vi "multiSineRT_inst.vi"() -> ()   [LabVIEW 2019]
uses:
  <vilib>/myRIO/Common/Instrument Driver Framework/myRIO v1.0/IRQ/typedefs/DI IRQ Type.ctl
  <vilib>/userDefined/High Color/nirio_resource_hc.ctl
  <vilib>/Platform/TimedLoop/XDataNode/timing_clust.ctl
  <vilib>/Platform/TimedLoop/XDataNode/nitl_modes.ctl
  <vilib>/Platform/TimedLoop/XDataNode/wakeup.ctl
  <vilib>/Utility/file.llb/Read Delimited Spreadsheet (DBL).vi
  rpm.vi
  ISR.vi
  <vilib>/myRIO/Common/Instrument Driver Framework/myRIO v1.0/IRQ/vis/myRIO v1.1 Register DI IRQ.vi
  <vilib>/Utility/file.llb/Write Delimited Spreadsheet (DBL).vi
  <vilib>/Utility/error.llb/Error Cluster From Error Code.vi
  <vilib>/myRIO/Common/Instrument Driver Framework/myRIO v1.0/PWM/vis/myRIO v1.0 Write PWM.vi
  <vilib>/myRIO/Common/Instrument Driver Framework/myRIO v1.0/IRQ/vis/myRIO v1.0 Reserve IRQ.vi
  <vilib>/myRIO/Common/Instrument Driver Framework/Utilities/vis/FPGA Ref Manager.vi
  <vilib>/myRIO/Common/Instrument Driver Framework/myRIO v1.0/myRIO v1.0 Close.vi
  <vilib>/myRIO/Express VI/IRQ/IRQ Express VI.xnode
  <vilib>/myRIO/Instrument Drivers/IRQ/IO IRQ/vis/myRIO Register DI IRQ.xnode
  <vilib>/myRIO/Common/Instrument Driver Framework/myRIO v1.0/IRQ/typedefs/Callback VI Ref.ctl
  <vilib>/platform/TimedLoop/XDataNode/XDataNode.xnode
  <vilib>/Platform/TimedLoop/XDataNode/XDNodeRunTimeDep.lvlib
  <vilib>/myRIO/Instrument Drivers/Onboard IO/PWM/PWM.lvlib
  <vilib>/Utility/Variable/NI_VariableUtilities.lvlib
  <vilib>/myRIO/Instrument Drivers/IRQ/IO IRQ/IO IRQ.lvlib
panel:
  out "g_p":dbl
  out "k_p":dbl
  out "error out (no error) 2":errorcluster
  out "p":dbl
  out "Commutations":i64
  out "RPM":dbl
  out "Iteration Duration":i64
  out "omega_vec":dbl[](array[numeric])
  out "Interrupt On":bool
  in  "RPM Inst Data":path=path "/tmp/log.csv"
  out "Omega":dbl[](graph)
  in  "error in (no error)":errorcluster
  out "Np":dbl
  out "ft":dbl
  in  "Input Data":path=path "/tmp/log.csv"
  in  "del_u":dbl=0.15
  in  "u_nominal":dbl=0.55
  out "Finished late":bool
  out "Acquisition State":bool
  in  "Run Time (s)":dbl
  in  "Sampling \nFrequency (Hz)":dbl
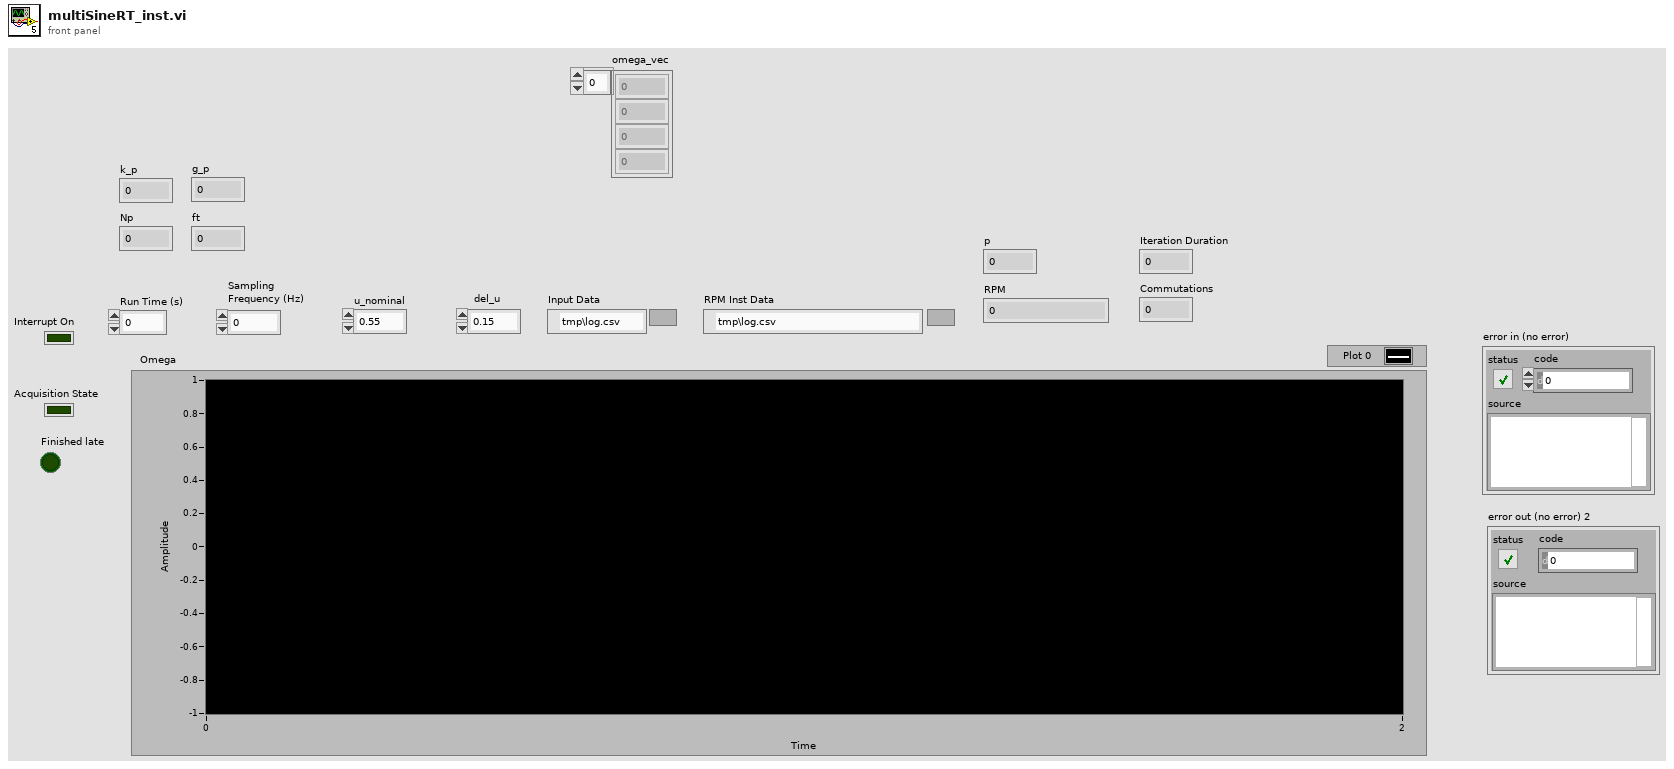
[diagram p1: front panel]
types:
  T1 = typedef "PWM.lvlib/PWM Reference.ctl" = cluster{"myRIO Reference":T2, "PWM Channels Enum":T6, "PWM Configuration":T7}
  T2 = typedef "myRIO Generic Hardware Reference.ctl" = cluster{"myRIO Model":T3, "myRIO Hardware Reference":T4}
  T3 = typedef "Hardware Version Enum.ctl" = enum16{"Unknown", "myRIO-1900", "myRIO-1950", "roboRIO", "NI ELVIS RIO CM", "ELVIS III"}
  T4 = typedef "myRIO v1.0 Reference.ctl" = cluster{"Generic FPGA Reference":T5, "Allow multiple opens":bool}
  T5 = typedef "Generic FPGA Reference.ctl" = refnum<k20>
  T6 = typedef "PWM Channels Enum.ctl" = enum16{"Not Connected", "C/PWM0", "C/PWM1", "A/PWM0", "A/PWM1", "A/PWM2", "A/PWM3", "A/PWM4", "A/PWM5", "A/PWM6", "A/PWM7", "A/PWM8", "A/PWM9", "A/PWM10", "A/PWM11", "A/PWM12", "A/PWM13", "A/PWM14", "A/PWM15", "A/PWM16", "A/PWM17", "A/PWM18", "A/PWM19", "B/PWM0", "B/PWM1", "B/PWM2", "B/PWM3", "B/PWM4", "B/PWM5", "B/PWM6", "B/PWM7", "B/PWM8", "B/PWM9", "B/PWM10", "B/PWM11", "B/PWM12", "B/PWM13", "B/PWM14", "B/PWM15", "B/PWM16", "B/PWM17", "B/PWM18", "B/PWM19", "PWM/PWM0", "PWM/PWM1", "PWM/PWM2", "PWM/PWM3", "PWM/PWM4", "PWM/PWM5", "PWM/PWM6", "PWM/PWM7", "PWM/PWM8", "PWM/PWM9"}
  T7 = typedef "PWM.lvlib/PWM Configuration.ctl" = cluster{"Frequency":dbl, "Duty Cycle":dbl}
  T8 = typedef "XDNodeRunTimeDep.lvlib/timing_clust.ctl" = cluster{"Expected End [f-1]":u64, "Actual End [f-1]":u64, "Finished Late? [f-1]":bool, "Expected End [i-1]":u64, "Actual End [i-1]":u64, "Finished Late? [i-1]":bool, "Expected Start [i]":u64, "Actual Start [i]":u64, "Expected Start [f]":u64, "Actual Start [f]":u64, "Source Name":string, "Structure Name":string, "Period":i64, "Deadline":i64, "Offset":i64, "Start":i64, "Priority":i32, "Timeout":i32, "Mode":T9, "Wakeup Reason":T10, "Error":errorcluster, "Source Type":string, "Secondary Source Type":string, "Global End Time":u64, "Global Start Time":u64, "Frame Duration":u64, "Iteration Duration":u64, "Assigned CPU":i32, "I/O Scan Engine Mode":u32}
  T9 = typedef "XDNodeRunTimeDep.lvlib/nitl_modes.ctl" = enum32{"No Change", "Process missed periods, maintain original phase", "Discard missed periods, maintain original phase", "Process missed periods, ignore original phase", "Discard missed periods, ignore original phase"}
  T10 = typedef "XDNodeRunTimeDep.lvlib/wakeup.ctl" = enum32{"Normal", "Aborted", "Asynchronous wakeup", "Timing source error", "Timed loop error", "Timeout"}
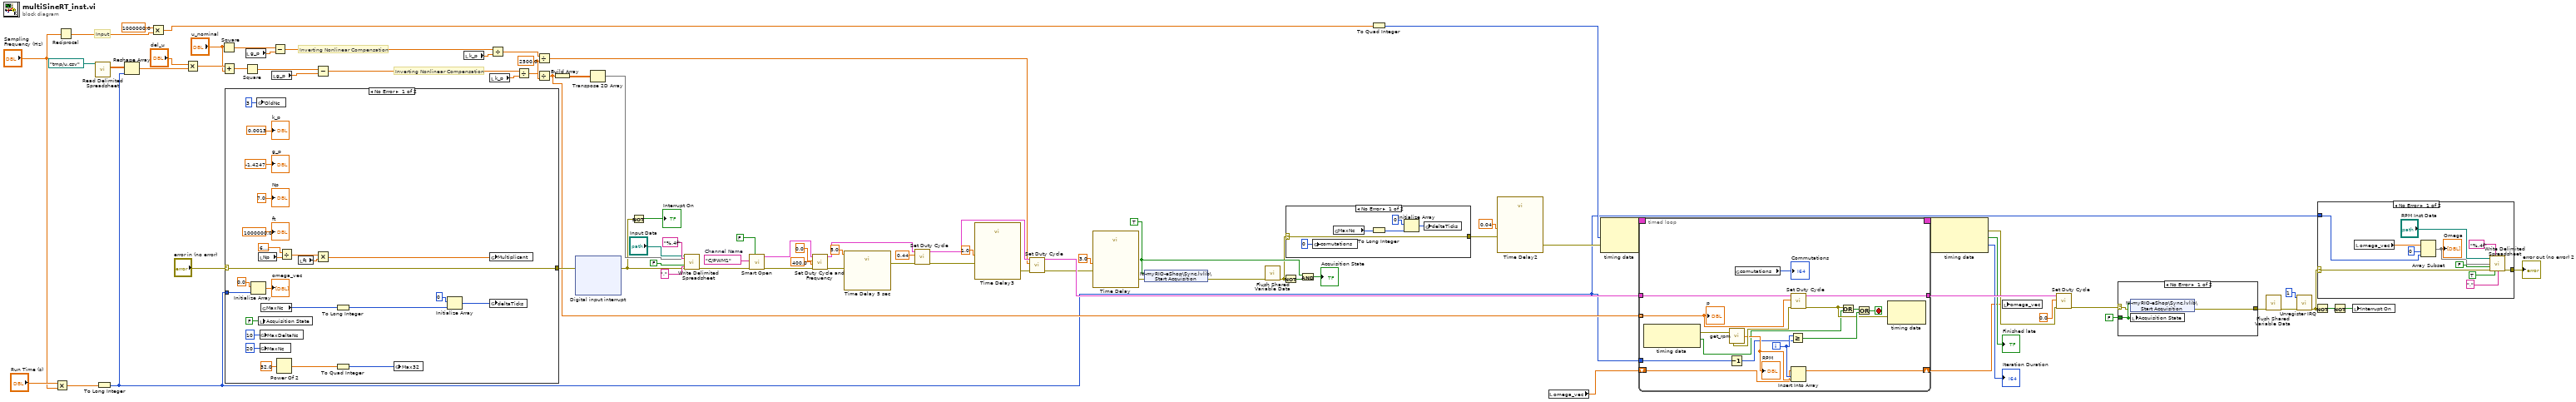
[diagram p0: block diagram]
diagram:
  w17 = 2500.0 ("y")
  w74 = tag "C/PWM1"  # Channel Name
  w53 = TRUE ("Acquisition State")
  # "Inverting Nonlinear Compensation"
  # "Inverting Nonlinear Compensation"
  # "Input"
  n1 = Multiply(x="Run Time (s)", y="Sampling \nFrequency (Hz)") -> (x*y=w76:dbl)
  n2 = Reciprocal(x="Sampling \nFrequency (Hz)") -> (1/x=w36:dbl)
  n3 = call-poly <vilib>:"Read Delimited Spreadsheet.vi"("file path (dialog if empty)"=path "/tmp/u.csv") -> ("all rows"=w63:dbl[][])  [unwired: 9 in, 5 out]
  n4 = To Long Integer(number=w76) -> (32bit integer=w13:i32)
  n5 = Reshape Array(w63, w13) -> (w62:dbl[])
  n6 = Multiply(x=1000000.0, y=w36) -> (x*y=w44:dbl)
  n7 = Multiply(x="del_u", y=w62) -> (x*y=w77:dbl[])
  n8 = Square(x="u_nominal") -> (x^2=w4:dbl)
  n9 = Add(x=w77, y="u_nominal") -> (x+y=w8:dbl[])
  n10 = case shown="No Error" "error in (no error)" {
    selector: "error in (no error)" -> [w105 w109]
    tunnel: [w105 w109] -> w50
    tunnel: w13 -> [w91 _]
    frame No Error {
      n11 = Initialize Array(0.0 ("element"), w91) -> (→"omega_vec":dbl[])
      n12 = global write "rpm.vi" "OldNc"(i64 3 ("MaxNc")) -> ()
      n13 = local read "Np"() -> (w101:dbl)
      n14 = local write "Acquisition State"(FALSE ("Acquisition State")) -> ()
      n15 = global write "rpm.vi" "MaxDeltaNc"(i64 10 ("MaxDeltaNc")) -> ()
      n16 = global write "rpm.vi" "MaxNc"(i64 20 ("MaxNc")) -> ()
      n17 = global read "rpm.vi" "MaxNc"() -> (w88:i64)
      n18 = Power Of 2(x=32.0) -> (2^x=w107:dbl)
      n19 = Divide(x=6.283185307179586, y=w101) -> (x/y=w100:dbl)
      n20 = local read "ft"() -> (w99:dbl)
      n21 = Multiply(x=w100, y=w99) -> (x*y=w108:dbl)
      n22 = To Long Integer(number=w88) -> (32bit integer=w87:i32)
      n23 = To Quad Integer(1:w107) -> (0:w98:i64)
      n24 = global write "rpm.vi" "Max32"(w98) -> ()
      n25 = Initialize Array(i64 0, w87) -> (w89:i64[])
      n26 = global write "rpm.vi" "Multiplicant"(w108) -> ()
      n27 = global write "rpm.vi" "deltaTicks"(w89) -> ()
      "Np" <- 7.0 ("Numeric")
      "ft" <- 1000000.0 ("ft")
      "k_p" <- 0.0013 ("k_p")
      "g_p" <- -1.4247 ("g_p")
    }
    frame Error {
    }
  }
  n28 = Square(x=w8) -> (x^2=w10:dbl[])
  n29 = local read "g_p"() -> (w5:dbl)
  n30 = local read "g_p"() -> (w11:dbl)
  n31 = Subtract(x=w4, y=w5) -> (x-y=w6:dbl)
  n32 = Subtract(x=w10, y=w11) -> (x-y=w12:dbl[])
  n33 = local read "k_p"() -> (w3:dbl)
  n34 = local read "k_p"() -> (w9:dbl)
  n35 = Divide(x=w6, y=w3) -> (x/y=w1:dbl)
  n36 = Divide(x=w12, y=w9) -> (x/y=w7:dbl[])
  n37 = Divide(x=w1, y=w17) -> (x/y=w18:dbl)
  n38 = Divide(x=w7, y=w17) -> (x/y=w19:dbl[])
  n39 = Build Array(w19) -> (w78:dbl[][])
  n40 = xnode "Digital input interrupt"("error in (no error)"=w50) -> ("error out"=w41:errorcluster)
  n41 = Transpose 2D Array(2D array=w78) -> (transposed array=w79:dbl[][])
  n42 = Not(x=w41) -> (.not. x?=→"Interrupt On":bool)
  n43 = call-poly <vilib>:"Write Delimited Spreadsheet.vi"("file path (dialog if empty)"="Input Data", "format (%.3f)"="%.4f", "2D data"=w79, "append to file? (new file:F)"=FALSE, "error in (no error)"=w41, "delimiter (\\t)"="," ("delimiter (\\t)")) -> ("error out"=w70:errorcluster)  [unwired: 8 in, 1 out]
  n44 = call <vilib>:"Smart Open.vi"("Allow multiple opens?"=FALSE, "error in (no error)"=w70, "Channel Name"=w74) -> ("error out"=w72:errorcluster, "PWM Ref Out"=w73:T1)  [unwired: 7 in]
  n45 = call <vilib>:"Set Duty Cycle and Frequency.vi"("error in (no error)"=w72, "Frequency [Hz]"=400.0, "Duty Cycle"=0.0, "PWM Ref In"=w73) -> ("error out"=w39:errorcluster, "PWM Ref Out"=w28:T1)  [unwired: 5 in]
  n46 = call "Time Delay 5 sec"("error in (no error)"=w39, "Delay Time (s)"=5.0) -> ("error out"=w29:errorcluster)  [unwired: 9 in]
  n47 = call <vilib>:"Set Duty Cycle.vi"("error in (no error)"=w29, "Duty Cycle"=0.44, "PWM Ref In"=w28) -> ("error out"=w32:errorcluster, "PWM Ref Out"=w26:T1)  [unwired: 6 in]
  n48 = call "Time Delay3"("error in (no error)"=w32, "Delay Time (s)"=1.0) -> ("error out"=w27:errorcluster)  [unwired: 9 in]
  n49 = call <vilib>:"Set Duty Cycle.vi"("error in (no error)"=w27, "Duty Cycle"=w18, "PWM Ref In"=w26) -> ("error out"=w37:errorcluster, "PWM Ref Out"=w38:T1)  [unwired: 6 in]
  n50 = call "Time Delay"("error in (no error)"=w37, "Delay Time (s)"=3.0) -> ("error out"=w65:errorcluster)  [unwired: 9 in]
  n51 = shared-variable "NI-myRIO-eShop\\Sync.lvlib\\Start Acquisition"(w53, error in=w65) -> (error out=w69:errorcluster)
  n52 = call <vilib>:"Flush Shared Variable Data.vi"("error in (no error)"=w69) -> ("error out"=w34:errorcluster)  [unwired: 10 in]
  n53 = Not(x=w34) -> (.not. x?=w33:bool)
  n54 = case shown="No Error" w34 {
    selector: w34 -> [w114 w116]
    tunnel: [w114 w116] -> w47
    frame No Error {
      n55 = global write "rpm.vi" "comutations"(i64 0 ("comutations")) -> ()
      n56 = global read "rpm.vi" "MaxNc"() -> (w111:i64)
      n57 = To Long Integer(number=w111) -> (32bit integer=w110:i32)
      n58 = Initialize Array(i64 0, w110) -> (w112:i64[])
      n59 = global write "rpm.vi" "deltaTicks"(w112) -> ()
    }
    frame Error {
    }
  }
  n60 = And(x=w53, y=w33) -> (x .and. y?=→"Acquisition State":bool)
  n61 = To Quad Integer(1:w44) -> (0:w43:i64)
  n62 = call "Time Delay2"("error in (no error)"=w47, "Delay Time (s)"=0.04) -> ("error out"=w60:errorcluster)  [unwired: 9 in]
  n63 = local read "omega_vec"() -> (w20:dbl[])
  n64 = node-c288(w43, w60) -> (w84:T8)  [unwired: 1 in]
  n65 = timed-loop {
    timing: w84 -> [_]
    timing-out: [_] -> w83
    tunnel: w19 -> [w128] mode=indexing
    tunnel: w38 -> [w133]
    tunnel: w13 -> [w118]
    tunnel: [w127] -> w56
    shift-right: [w120] -> w16
    shift-left: w20 -> [w121]
    i -> [w123]
    stop <- w132 stop-if-true
    n66 = node-c288() -> (w126:errorcluster, w122:bool)  [unwired: 1 in]
    n67 = Decrement(x=w118) -> (x-1=w117:i32)
    n68 = call "get_rpm.vi"("error in (no error)"=w126) -> ("RPM"=w124:dbl, "error out"=w125:errorcluster)
    "RPM" <- w124
    n69 = global read "rpm.vi" "comutations"() -> (→"Commutations":i64)
    n70 = Greater Or Equal?(x=w123, y=w117) -> (x >= y?=w130:bool)
    n71 = call <vilib>:"Set Duty Cycle.vi"("error in (no error)"=w125, "Duty Cycle"=w128, "PWM Ref In"=w133) -> ("error out"=w129:errorcluster, "PWM Ref Out"=w127:T1)  [unwired: 6 in]
    n72 = Insert Into Array(array=w121, index=w123, new element=w124) -> (w120:dbl[])
    n73 = Or(x=w129, y=w122) -> (x .or. y?=w131:bool)
    n74 = Or(x=w131, y=w130) -> (x .or. y?=w132:bool)
    n75 = node-c288(w129) -> ()  [unwired: 1 in, 1 out]
    "p" <- w128
  }
  n76 = node-c288(w83) -> (w55:errorcluster, →"Finished late":bool, →"Iteration Duration":i64)
  n77 = local write "omega_vec"(w16) -> ()
  n78 = call <vilib>:"Set Duty Cycle.vi"("error in (no error)"=w55, "Duty Cycle"=0.0, "PWM Ref In"=w56) -> ("error out"=w23:errorcluster)  [unwired: 6 in, 1 out]
  n79 = case shown="No Error" w23 {
    selector: w23 -> [w140 w143]
    tunnel: [w142 w143] -> w68
    tunnel: FALSE ("Start Acquisition") -> [w141 _]
    frame No Error {
      n80 = shared-variable "NI-myRIO-eShop\\Sync.lvlib\\Start Acquisition"(w141, error in=w140) -> (error out=w142:errorcluster)
      n81 = local write "Acquisition State"(w141) -> ()
    }
    frame Error {
    }
  }
  n82 = call <vilib>:"Flush Shared Variable Data.vi"("error in (no error)"=w68) -> ("error out"=w48:errorcluster)  [unwired: 10 in]
  n83 = call <vilib>:"Unregister IRQ.vi"("error in (no error)"=w48, "IRQ Number"=u8 1) -> ("error out"=w15:errorcluster)  [unwired: 9 in]
  n84 = Not(x=w15) -> (.not. x?=w25:bool)
  n85 = case shown="No Error" w15 {
    selector: w15 -> [w149 w155]
    tunnel: [w148 w155] -> w14
    tunnel: w13 -> [w144 _]
    frame No Error {
      n86 = local read "omega_vec"() -> (w147:dbl[])
      n87 = Array Subset(array=w147, index=0, length=w144) -> (w146:dbl[])
      "Omega" <- w146
      n88 = call-poly <vilib>:"Write Delimited Spreadsheet.vi"("file path (dialog if empty)"="RPM Inst Data", "format (%.3f)"="%.4f", "1D data"=w146, "append to file? (new file:F)"=FALSE, "error in (no error)"=w149, "transpose? (no:F)"=TRUE, "delimiter (\\t)"="," ("delimiter (\\t)")) -> ("error out"=w148:errorcluster)  [unwired: 7 in, 1 out]
    }
    frame Error {
    }
  }
  "error out (no error) 2" <- w14
  n89 = Not(x=w25) -> (.not. x?=w24:bool)
  n90 = local write "Interrupt On"(w24) -> ()
